vi "read 2b prefixed string.vi"(8 "error in (no error)":errorcluster, 11 "TCP Network Connection in":refnum<k5>) -> (0 "error out":errorcluster, 2 "data out":string, 3 "TCP Network Connection out":refnum<k5>)   [LabVIEW 2020]
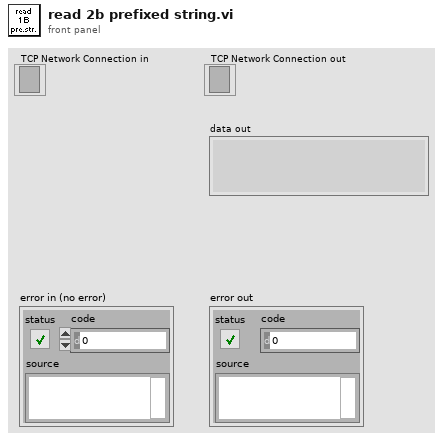
[diagram p1: front panel]
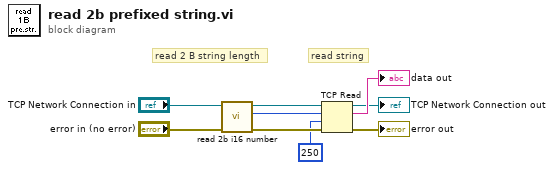
[diagram p0: block diagram]
diagram:
  # "read string"
  # "read 2 B string length"
  n1 = call "read 2b i16 number.vi"("error in (no error)"="error in (no error)", "TCP Network Connection in"="TCP Network Connection in") -> ("error out"=w3:errorcluster, "number"=w5:i16, "TCP Network Connection out"=w2:refnum<k5>)  [unwired: 7 in]
  n2 = TCP Read(connection ID=w2, bytes to read=w5, error in (no error)=w3, 9:250 ("timeout ms (25000)")) -> (connection ID out=→"TCP Network Connection out":refnum<k5>, data out=→"data out":string, error out=→"error out":errorcluster)  [unwired: 1 in]
